vi "Serial Write.vi"(8 "error in (no error)":errorcluster {"code" format="%.0x"}, 10 "Write Buffer (\"\")":string, 11 "VISA resource name":refnum<visa-resource-name>) -> (0 "error out":errorcluster {"code" format="%.0x"}, 2 "Return Count":u32, 3 "VISA resource name out":refnum<visa-resource-name>)   [LabVIEW 2021, in "Lake Shore Cryotronics 331.lvlib"]
doc: "This VI appends the carriage return, line feed characters \"\\r\\n\" to the end of the input string and writes the new string to the instrument."
uses:
  <instrlib>/Lake Shore Cryotronics 331/Lake Shore Cryotronics 331.lvlib
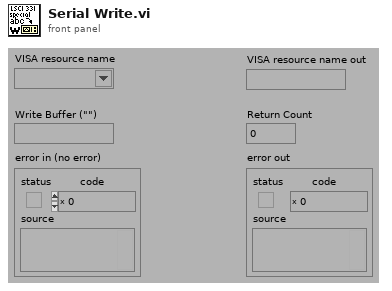
[diagram p1: front panel]
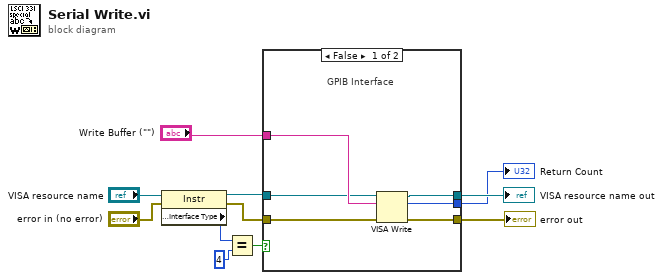
[diagram p0: block diagram]
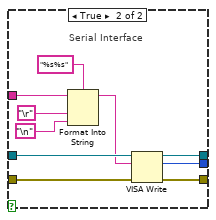
[diagram p2: hidden frame]
diagram:
  n1 = property class="Instr"(reference="VISA resource name", error in="error in (no error)") -> (reference out=w4:refnum<visa-resource-name>, error out=w5:errorcluster, "Interface Information:Interface Type"=w2:u16)
  n2 = Equal?(x=w2, y=4) -> (x = y?=w1:bool)
  n3 = case shown="False" w1 {
    tunnel: [w14 w27] -> w11
    tunnel: [w12 w26] -> w10
    tunnel: [w13 w25] -> w9
    tunnel: w4 -> [w16 w24]
    tunnel: w5 -> [w15 w23]
    tunnel: "Write Buffer (\"\")" -> [w17 w22]
    frame False {
      # "GPIB Interface"
      n4 = VISA Write(VISA resource name=w16, write buffer=w17, error in (no error)=w15) -> (VISA resource name out=w12:refnum<visa-resource-name>, return count=w13:u32, error out=w14:errorcluster)
    }
    frame True {
      # "Serial Interface"
      n5 = Format Into String(format string="%s%s", initial string=w22, "\r", "\n") -> (resulting string=w18:string)  [unwired: 1 in, 1 out]
      n6 = VISA Write(VISA resource name=w24, write buffer=w18, error in (no error)=w23) -> (VISA resource name out=w26:refnum<visa-resource-name>, return count=w25:u32, error out=w27:errorcluster)
    }
  }
  "VISA resource name out" <- w10
  "error out" <- w11
  "Return Count" <- w9
